vi "Prep for GETCONF.vi"(8 "Error In":errorcluster, 10 "Parameter and Value":string="SETCONF=SMUResourceName[[CONFPARAM]]=SMU") -> (0 "Error Out":errorcluster, 2 "GETCONF Parameter":string="GETCONF=SMUResourceName")   [LabVIEW 2019]
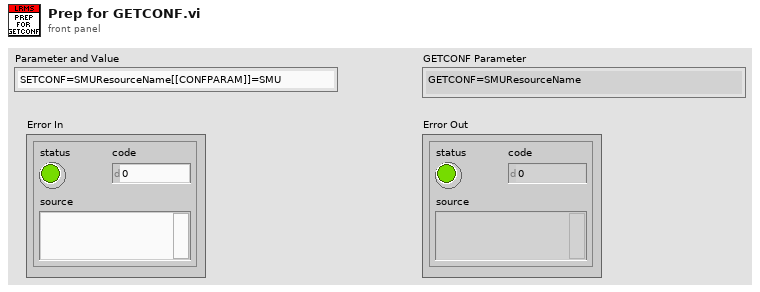
[diagram p1: front panel]
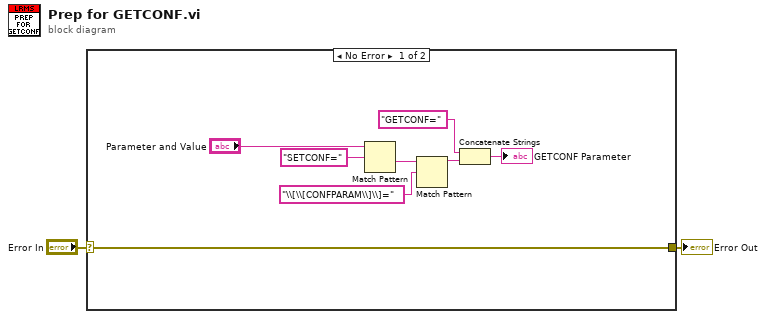
[diagram p0: block diagram]
diagram:
  n1 = case shown="No Error" "Error In" {
    selector: "Error In" -> [w3 w11]
    tunnel: [w3 w11] -> w1
    frame No Error {
      n2 = Match Pattern(string="Parameter and Value", regular expression="SETCONF=" ("default value 1")) -> (after substring=w6:string)  [unwired: 1 in, 3 out]
      n3 = Match Pattern(string=w6, regular expression="\\[\\[CONFPARAM\\]\\]=" ("default value 1")) -> (before substring=w4:string)  [unwired: 1 in, 3 out]
      n4 = Concatenate Strings("GETCONF=" ("default value 1"), w4) -> (→"GETCONF Parameter":string)
    }
    frame Error {
    }
  }
  "Error Out" <- w1
